vi "appendError.vi"(8 "error in (no error)":errorcluster, 9 "Boolean":bool, 10 "code":i32, 11 "String":string) -> (0 "error out":errorcluster)   [LabVIEW 2015]
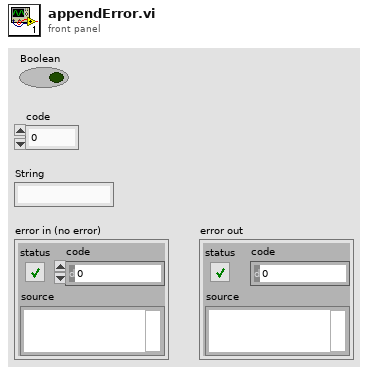
[diagram p1: front panel]
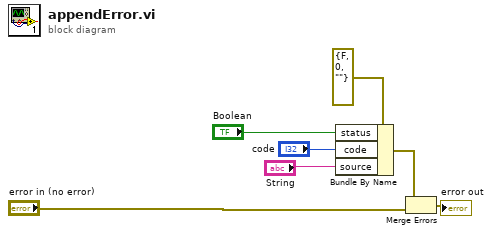
[diagram p0: block diagram]
diagram:
  n1 = Bundle By Name(cluster=errorcluster {"status"=FALSE, "code"=0, "source"=""} ("error in (no error)"), "status"="Boolean", "code"="code", "source"="String") -> (w1:errorcluster)
  n2 = Merge Errors(w1, "error in (no error)") -> (→"error out":errorcluster)
